vi "Update Connected Client ListBox.vi"(8 "error in (no error)":errorcluster, 11 "Function in":refnum<class "Function.lvclass">) -> (0 "error out":errorcluster, 3 "Function out":refnum<class "Function.lvclass">)   [LabVIEW 2016, in "Function Actor.lvlib" / "Function.lvclass"]
uses:
  <userlib>/Common Components/Function Actor/Function.lvclass
  <userlib>/Common Components/Function Actor/Function.lvclass/Function.ctl
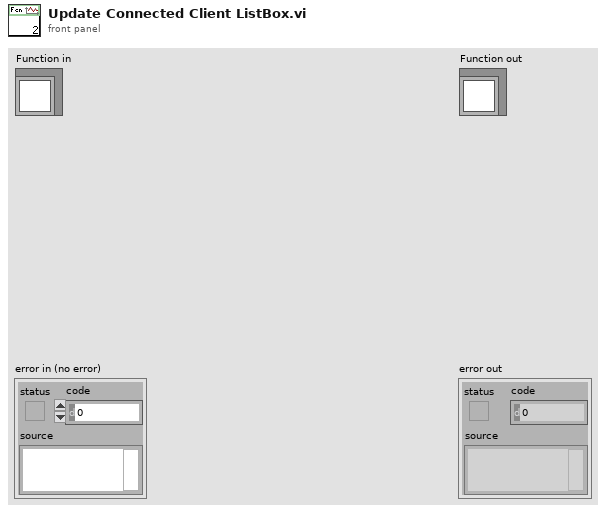
[diagram p1: front panel]
types:
  T1 = typedef "Common.lvlib/Connection Cluster.ctl" = cluster{"GUID":string, "Connected Client Cluster":T2}
  T2 = typedef "Common.lvlib/Connected Client Cluster.ctl" = cluster{"IP Address":string, "Username":string, "Access Level":string}
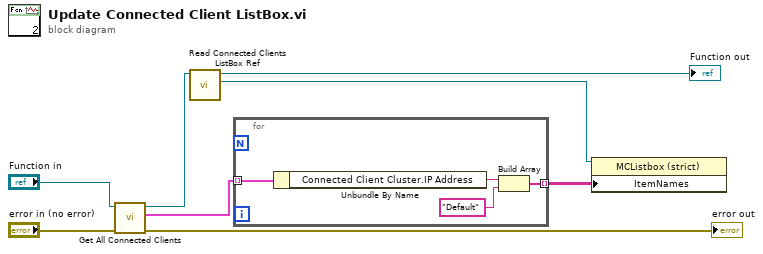
[diagram p0: block diagram]
diagram:
  n1 = call <userlib>:"Get All Connected Clients.vi"("error in (no error)"="error in (no error)", "Function in"="Function in") -> ("error out"=→"error out":errorcluster, "Array of Connected Clients"=w4:T1[], "Function out"=w5:refnum<class "Function.lvclass">)  [unwired: 7 in]
  n2 = call <userlib>:"Read Connected Clients ListBox Ref.vi"("Function in"=w5) -> ("Connected Clients"=w2:refnum<vi>, "Function out"=→"Function out":refnum<class "Function.lvclass">)  [unwired: 9 in]
  n3 = for {
    tunnel: w4 -> [w12] mode=indexing
    tunnel: [w9] -> w1 mode=indexing
    n4 = Unbundle By Name(w12) -> ("Connected Client Cluster.IP Address"=w11:string)
    n5 = Build Array(w11, "Default" ("element")) -> (w9:string[])
  }
  n6 = property class="MCListbox (strict)"(reference=w2, "ItemNames"=w1) -> ()  [unwired: 1 in, 2 out]
